vi "hw3.2.vi"() -> ()   [LabVIEW 2014]
panel:
  out "Waveform Graph":dbl[](graph)
  out "output array":dbl[](array[numeric])
  out "Array":dbl[](array[numeric])
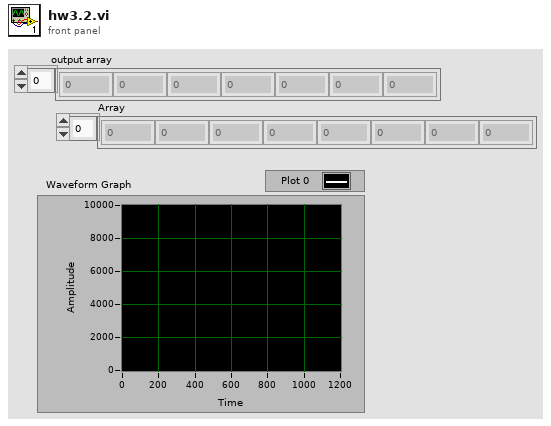
[diagram p1: front panel]
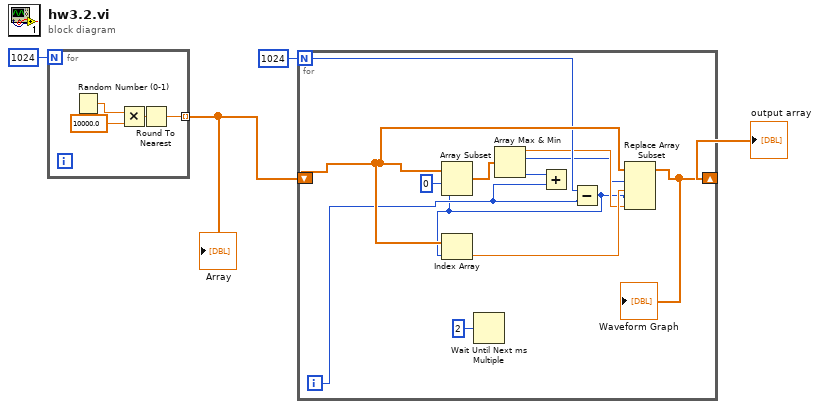
[diagram p0: block diagram]
diagram:
  n1 = for {
    N: 1024 -> [_]
    tunnel: [w5] -> w3 mode=indexing
    n2 = Random Number (0-1)() -> (number: 0 to 1=w8:dbl)
    n3 = Multiply(x=w8, y=10000.0) -> (x*y=w6:dbl)
    n4 = Round To Nearest(number=w6) -> (nearest integer value=w5:dbl)
  }
  "Array" <- w3
  n5 = for {
    N: 1024 -> [w14]
    shift-right: [w16] -> w1
    shift-left: w3 -> [w17]
    i -> [w11]
    n6 = Wait Until Next ms Multiple(millisecond multiple=u32 2) -> ()  [unwired: 1 out]
    n7 = Subtract(x=w14, y=w11) -> (x-y=w9:i32)
    n8 = Array Subset(array=w17, index=0, length=w9) -> (w20:dbl[])
    n9 = Index Array(array=w17, index=w9) -> (element=w18:dbl)
    n10 = Array Max & Min(array=w20) -> (max value=w13:dbl, max index (indices)=w12:i32, min index (indices)=w19:i32)  [unwired: 1 out]
    n11 = Add(x=w19, y=w11) -> ()  [unwired: 1 out]
    n12 = Replace Array Subset(array=w17, new element #1=w18, index #1=w12, new element #2=w13, index #2=w9) -> (w16:dbl[])
    "Waveform Graph" <- w16
  }
  "output array" <- w1
